vi "TDMS Write.vi"   [LabVIEW 2017]
types:
  T1 = enum16{"open", "open or create", "create or replace", "create", "open (read-only)"}
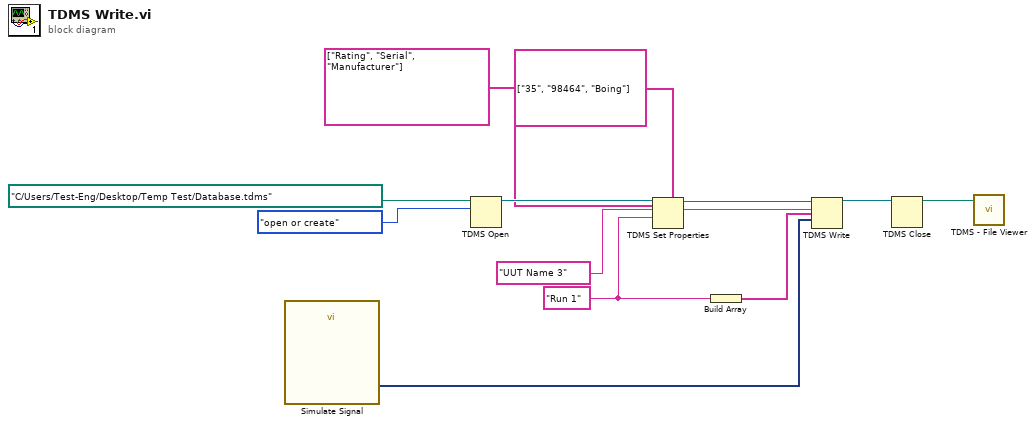
[diagram p0: block diagram]
diagram:
  w2 = "Run 1" ("channel name")
  n1 = call "Simulate Signal"() -> ("Sine"=w11:dynamicdata)  [unwired: 14 in, 1 out]
  n2 = TDMS Open(10:T1."open or create" ("operation (0:open)"), 11:path "C:/Users/Test-Eng/Desktop/Temp Test/Database.tdms" ("file path")) -> (3:w9:refnum<k34>)  [unwired: 5 in, 1 out]
  n3 = TDMS Set Properties(5:string[] ["35", "98464", "Boing"] ("property names"), 7:string[] ["Rating", "Serial", "Manufacturer"] ("property names"), 9:w2, 10:"UUT Name 3" ("group name in (Untitled)"), 11:w9) -> (2:w7:string, 3:w8:refnum<k34>)  [unwired: 1 in, 2 out]
  n4 = Build Array(w2) -> (w1:string[])
  n5 = TDMS Write(0:w8, 5:w7, 7:w1, 9:w11) -> (4:w3:refnum<k34>)  [unwired: 2 in, 3 out]
  n6 = TDMS Close(11:w3) -> (3:w10:path)  [unwired: 1 in, 1 out]
  n7 = call <vilib>:"TDMS - File Viewer.vi"("file path"=w10) -> ()  [unwired: 5 in, 2 out]
